vi "readU48.vi"(8 "error in (no error)":errorcluster, 11 "ModbusBuffer in":refnum<class "ModbusBuffer.lvclass">) -> (0 "error out":errorcluster, 2 "Output":u64, 3 "ModbusBuffer out":refnum<class "ModbusBuffer.lvclass">)   [LabVIEW 2016, in "RTModbus.lvlib" / "ModbusBuffer.lvclass"]
uses:
  ModbusBuffer.lvclass
  ModbusBuffer.lvclass/ModbusBuffer.ctl
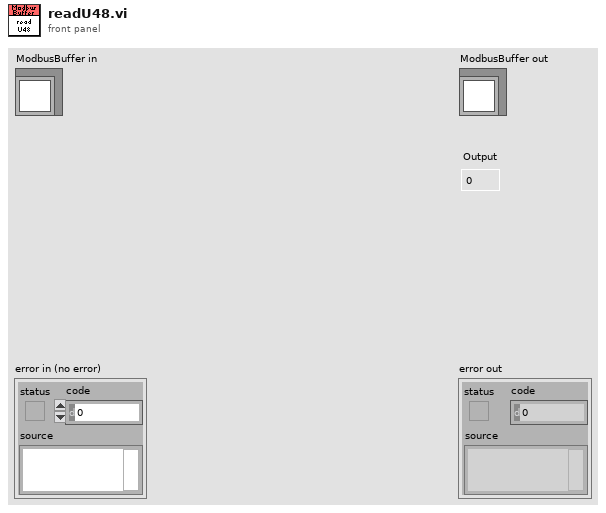
[diagram p1: front panel]
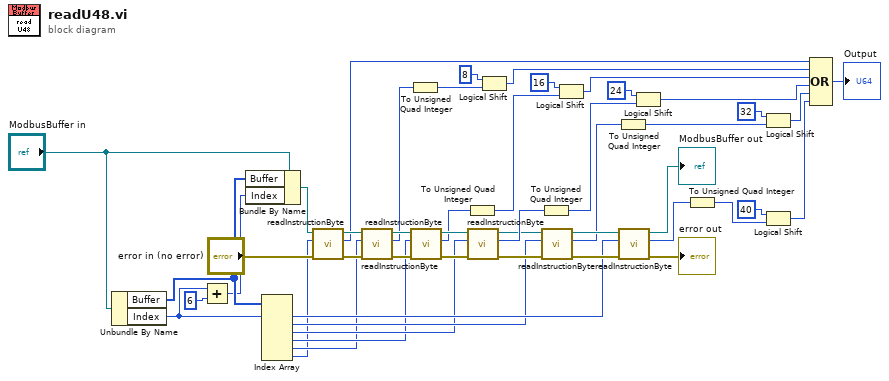
[diagram p0: block diagram]
diagram:
  n1 = Unbundle By Name("ModbusBuffer in") -> ("Buffer"=w46:u16[], "Index"=w43:i32)
  n2 = Add(x=w43, y=6) -> (x+y=w41:i32)
  n3 = Bundle By Name(cluster="ModbusBuffer in", "Buffer"=w46, "Index"=w41) -> (w45:refnum<class "ModbusBuffer.lvclass">)
  n4 = Index Array(array=w46, index #1=w43) -> (element #1=w6:u16, element #2=w5:u16, element #3=w4:u16, element #4=w3:u16, element #5=w2:u16, element #6=w1:u16)  [unwired: 5 in]
  n5 = call "readInstructionByte.vi"("error in (no error)"="error in (no error)", "Instruction"=w1, "ModbusBuffer in"=w45) -> ("error out"=w38:errorcluster, "Output"=w39:u8, "ModbusBuffer out"=w40:refnum<class "ModbusBuffer.lvclass">)  [unwired: 6 in]
  n6 = call "readInstructionByte.vi"("error in (no error)"=w38, "Instruction"=w2, "ModbusBuffer in"=w40) -> ("error out"=w32:errorcluster, "Output"=w26:u8, "ModbusBuffer out"=w34:refnum<class "ModbusBuffer.lvclass">)  [unwired: 6 in]
  n7 = To Unsigned Quad Integer(1:w26) -> (0:w25:u64)
  n8 = call "readInstructionByte.vi"("error in (no error)"=w32, "Instruction"=w3, "ModbusBuffer in"=w34) -> ("error out"=w31:errorcluster, "Output"=w24:u8, "ModbusBuffer out"=w33:refnum<class "ModbusBuffer.lvclass">)  [unwired: 6 in]
  n9 = To Unsigned Quad Integer(1:w24) -> (0:w23:u64)
  n10 = call "readInstructionByte.vi"("error in (no error)"=w31, "Instruction"=w4, "ModbusBuffer in"=w33) -> ("error out"=w14:errorcluster, "Output"=w22:u8, "ModbusBuffer out"=w16:refnum<class "ModbusBuffer.lvclass">)  [unwired: 6 in]
  n11 = Logical Shift(y=i16 8, x=w25) -> (x << y=w36:u64)
  n12 = To Unsigned Quad Integer(1:w22) -> (0:w21:u64)
  n13 = call "readInstructionByte.vi"("error in (no error)"=w14, "Instruction"=w5, "ModbusBuffer in"=w16) -> ("error out"=w13:errorcluster, "Output"=w12:u8, "ModbusBuffer out"=w15:refnum<class "ModbusBuffer.lvclass">)  [unwired: 6 in]
  n14 = Logical Shift(y=i16 16, x=w23) -> (x << y=w27:u64)
  n15 = To Unsigned Quad Integer(1:w12) -> (0:w20:u64)
  n16 = call "readInstructionByte.vi"("error in (no error)"=w13, "Instruction"=w6, "ModbusBuffer in"=w15) -> ("error out"=→"error out":errorcluster, "Output"=w11:u8, "ModbusBuffer out"=→"ModbusBuffer out":refnum<class "ModbusBuffer.lvclass">)  [unwired: 6 in]
  n17 = Logical Shift(y=i16 24, x=w21) -> (x << y=w28:u64)
  n18 = To Unsigned Quad Integer(1:w11) -> (0:w17:u64)
  n19 = Logical Shift(y=i16 32, x=w20) -> (x << y=w10:u64)
  n20 = Logical Shift(y=i16 40, x=w17) -> (x << y=w9:u64)
  n21 = Compound Arithmetic op=OR(w39, w36, w27, w28, w10, w9) -> (→"Output":u64)
